vi "DriveJoystickButtonMapping.vi"(11 "drive joystick buttons":bool[](array[boolean])) -> (3 "DriveJoystickButtonMapping":T1, 4 "drive joystick buttons indicator":bool[](array[boolean]))   [LabVIEW 2018]
uses:
  DriveJoystickButtonMapping.ctl
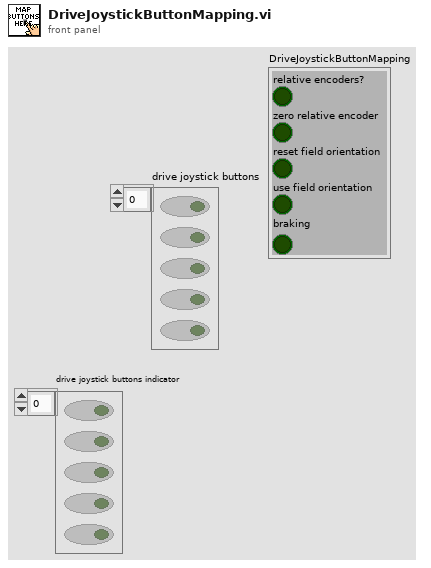
[diagram p1: front panel]
types:
  T1 = typedef "DriveJoystickButtonMapping.ctl" = cluster{"relative encoders?":bool, "zero relative encoder":bool, "reset field orientation":bool, "use field orientation":bool, "braking":bool}
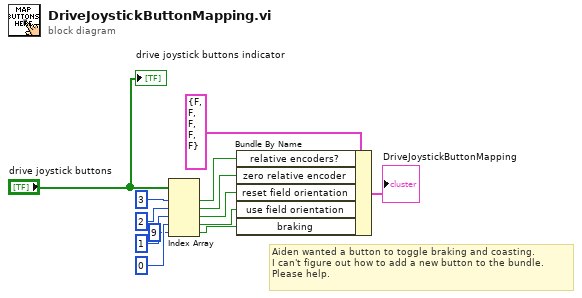
[diagram p0: block diagram]
diagram:
  # "Aiden wanted a button to toggle braking and coasting.\nI can't figure out how to add a new button to the bundle.\nPlease help."
  n1 = Index Array(array="drive joystick buttons", index #1=3 ("index"), index #2=2 ("index"), index #3=1 ("index"), index #4=0 ("index"), index #5=9 ("index")) -> (element #1=w7:bool, element #2=w6:bool, element #3=w5:bool, element #4=w4:bool, element #5=w1:bool)
  n2 = Bundle By Name(cluster=T1 {"relative encoders?"=FALSE, "zero relative encoder"=FALSE, "reset field orientation"=FALSE, "use field orientation"=FALSE, "braking"=FALSE} ("DriveJoystickButtonMapping"), "relative encoders?"=w7, "zero relative encoder"=w6, "reset field orientation"=w5, "use field orientation"=w4, "braking"=w1) -> (→"DriveJoystickButtonMapping":T1)
  "drive joystick buttons indicator" <- "drive joystick buttons"
